vi "KEVIN GET USERS ITEMS.vi"(10 "BYU ID # IN":string, 11 "connection reference in":T3) -> (2 "DATA OUT":T2, 3 "connection reference out":T3)   [LabVIEW 2019]
uses:
  <vilib>/addons/database/Connection.llb/Conn ObjectReference.ctl
  Controls/Table Data Types/Inventory Data Type.ctl
  <vilib>/addons/database/Auxilliary.llb/DB Tools Cursor Type.ctl
  <vilib>/addons/database/Connection.llb/Conn Execute.vi
  <vilib>/addons/database/Recordset.llb/Rec Fetch Recordset Data (R).vi
  <vilib>/addons/database/Recordset.llb/Rec Destroy - Connection.vi
  <vilib>/addons/database/_DB Variant To Data/Database Variant To Data.xnode
  <vilib>/addons/database/NI_Database_API.lvlib
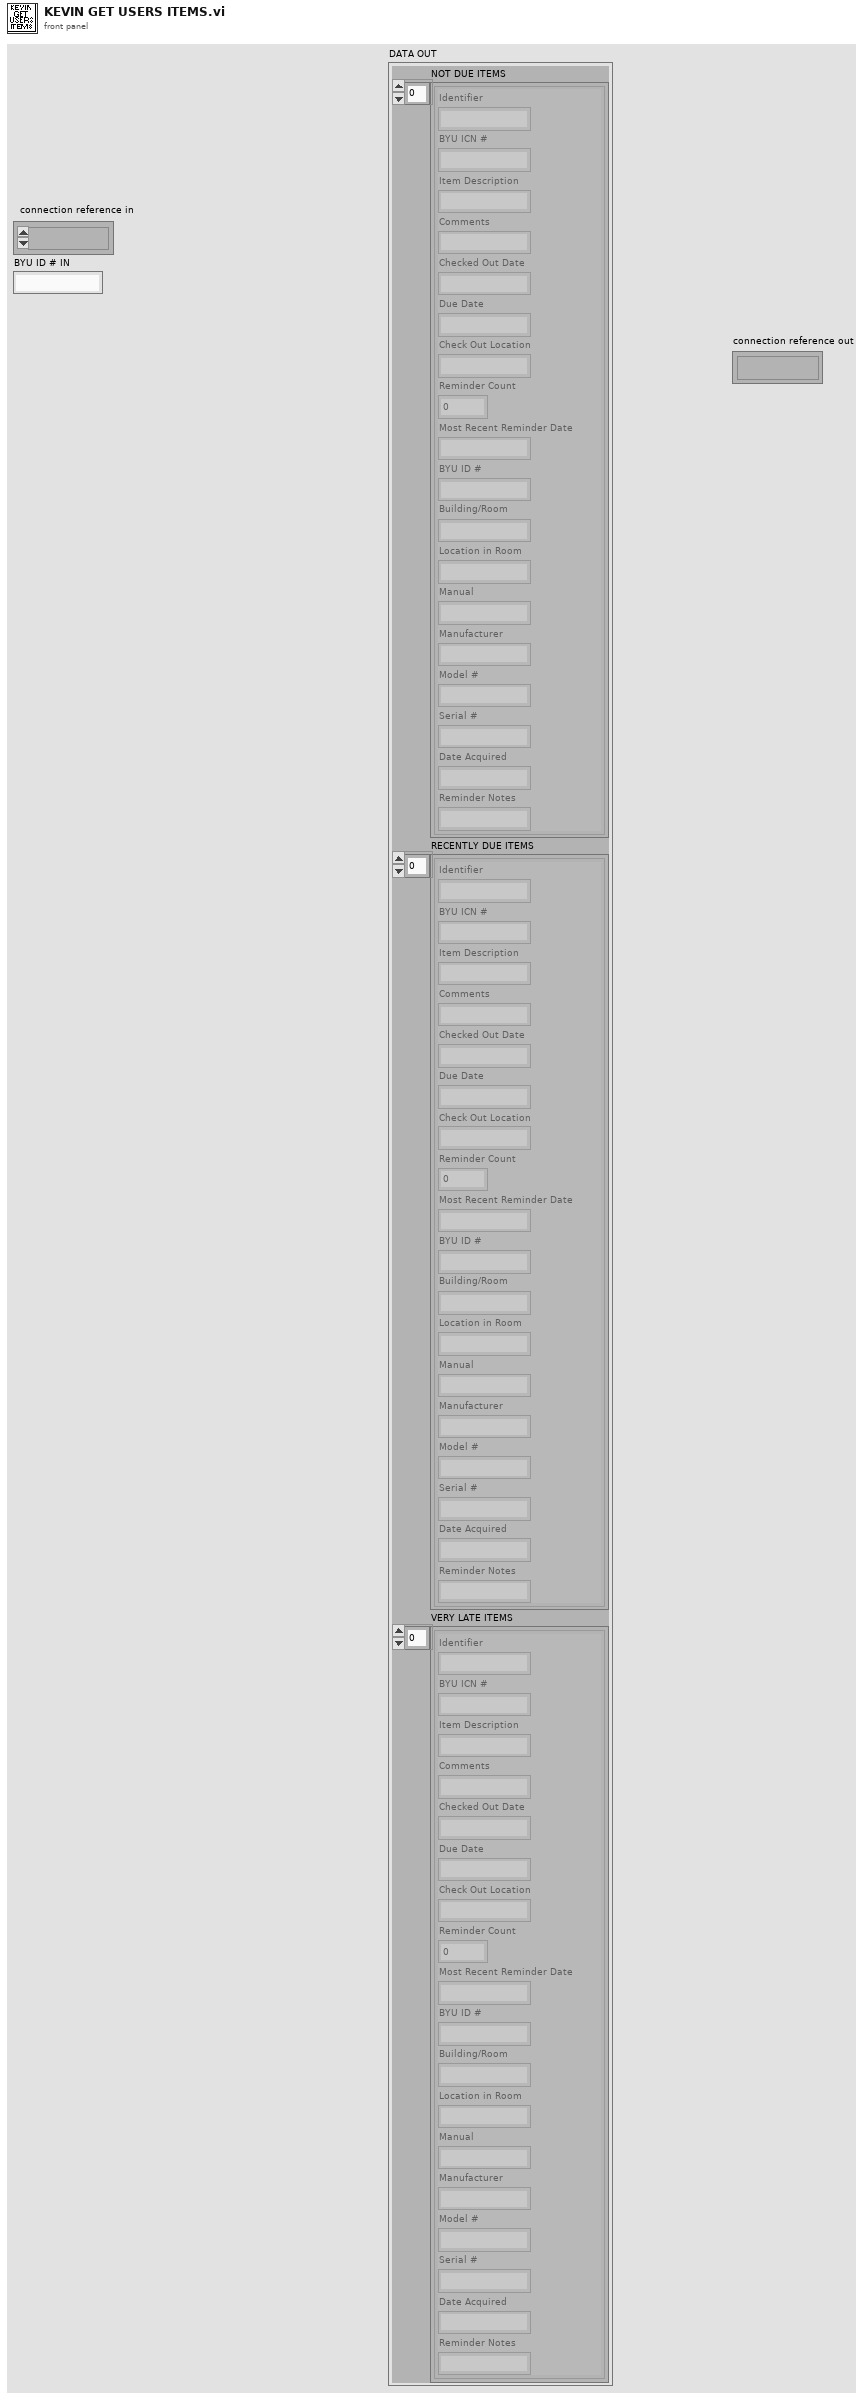
[diagram p1: front panel]
types:
  T1 = typedef "Inventory Data Type.ctl" = cluster{"Identifier":string, "BYU ICN #":string, "Item Description":string, "Comments":string, "Checked Out Date":string, "Due Date":string, "Check Out Location":string, "Reminder Count":i32, "Most Recent Reminder Date":string, "BYU ID #":string, "Building/Room":string, "Location in Room":string, "Manual":string, "Manufacturer":string, "Model #":string, "Serial #":string, "Date Acquired":string, "Reminder Notes":string}
  T2 = cluster{"NOT DUE ITEMS":T1[], "RECENTLY DUE ITEMS":T1[], "VERY LATE ITEMS":T1[]}
  T3 = typedef "NI_Database_API.lvlib/Conn ObjectReference.ctl" = refnum<k1>
  T4 = typedef "NI_Database_API.lvlib/DB Tools Cursor Type.ctl" = enum16{"forward-only", "keyset", "dynamic", "static"}
  T5 = typedef "NI_Database_API.lvlib/Rec ObjectReference.ctl" = refnum<k1>
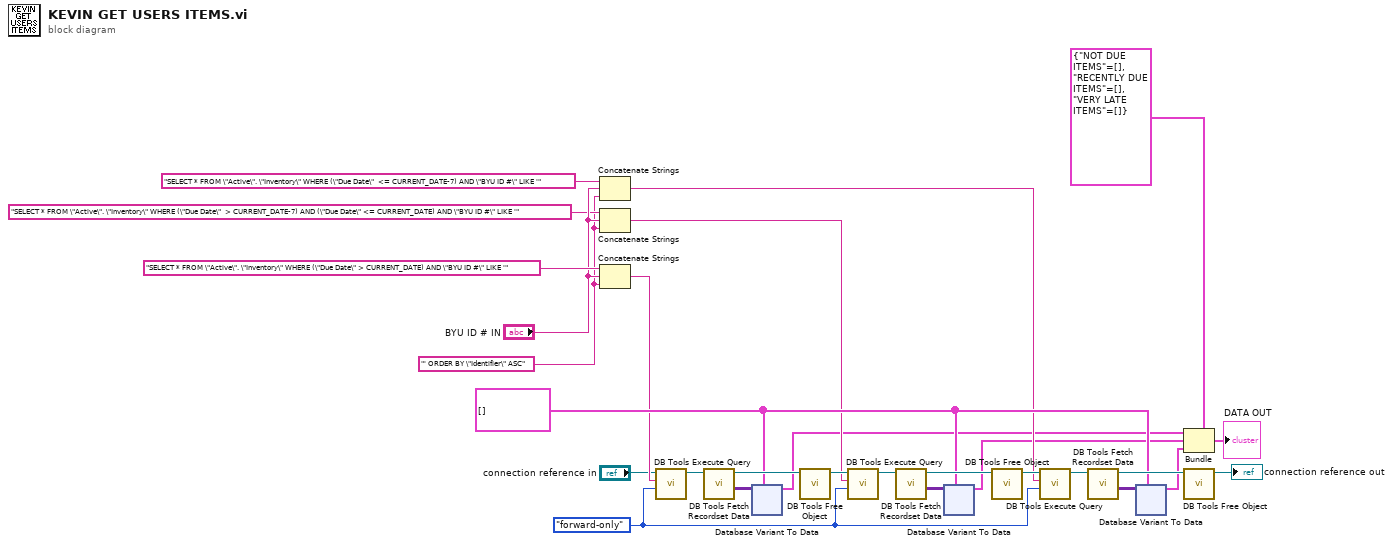
[diagram p0: block diagram]
diagram:
  w13 = DB_Tools_Cursor_Type."forward-only" ("cursor type")
  w7 = "' ORDER BY \"Identifier\" ASC"
  w15 = T1[] [] ("Array")
  n1 = Concatenate Strings("SELECT * FROM \"Active\". \"Inventory\" WHERE (\"Due Date\"  <= CURRENT_DATE-7) AND \"BYU ID #\" LIKE '", "BYU ID # IN", w7) -> (w11:string)
  n2 = Concatenate Strings("SELECT * FROM \"Active\". \"Inventory\" WHERE (\"Due Date\"  > CURRENT_DATE-7) AND (\"Due Date\" <= CURRENT_DATE) AND \"BYU ID #\" LIKE '", "BYU ID # IN", w7) -> (w12:string)
  n3 = Concatenate Strings("SELECT * FROM \"Active\". \"Inventory\" WHERE (\"Due Date\" > CURRENT_DATE) AND \"BYU ID #\" LIKE '", "BYU ID # IN", w7) -> (w14:string)
  n4 = call-poly <vilib>:"DB Tools Execute Query.vi"("cursor type"=w13, "SQL query"=w14, "connection reference"="connection reference in") -> ("recordset reference"=w24:T5)  [unwired: 5 in, 1 out]
  n5 = call-poly <vilib>:"DB Tools Fetch Recordset Data.vi"("recordset reference"=w24) -> ("recordset data"=w26:variant[][], "recordset reference out"=w25:T5)  [unwired: 4 in, 1 out]
  n6 = xnode "Database Variant To Data"("database variant"=w26, "type"=w15) -> ("data"=w4:T1[])  [unwired: 1 in, 1 out]
  n7 = call-poly <vilib>:"DB Tools Free Object.vi"("recordset reference"=w25) -> ("connection reference"=w20:T3)  [unwired: 9 in, 1 out]
  n8 = call-poly <vilib>:"DB Tools Execute Query.vi"("cursor type"=w13, "SQL query"=w12, "connection reference"=w20) -> ("recordset reference"=w23:T5)  [unwired: 5 in, 1 out]
  n9 = call-poly <vilib>:"DB Tools Fetch Recordset Data.vi"("recordset reference"=w23) -> ("recordset data"=w21:variant[][], "recordset reference out"=w22:T5)  [unwired: 4 in, 1 out]
  n10 = xnode "Database Variant To Data"("database variant"=w21, "type"=w15) -> ("data"=w3:T1[])  [unwired: 1 in, 1 out]
  n11 = call-poly <vilib>:"DB Tools Free Object.vi"("recordset reference"=w22) -> ("connection reference"=w16:T3)  [unwired: 9 in, 1 out]
  n12 = call-poly <vilib>:"DB Tools Execute Query.vi"("cursor type"=w13, "SQL query"=w11, "connection reference"=w16) -> ("recordset reference"=w17:T5)  [unwired: 5 in, 1 out]
  n13 = call-poly <vilib>:"DB Tools Fetch Recordset Data.vi"("recordset reference"=w17) -> ("recordset data"=w19:variant[][], "recordset reference out"=w18:T5)  [unwired: 4 in, 1 out]
  n14 = xnode "Database Variant To Data"("database variant"=w19, "type"=w15) -> ("data"=w2:T1[])  [unwired: 1 in, 1 out]
  n15 = Bundle(cluster=T2 {"NOT DUE ITEMS"=[], "RECENTLY DUE ITEMS"=[], "VERY LATE ITEMS"=[]} ("EMAIL ITEMS"), "NOT DUE ITEMS"=w4, "RECENTLY DUE ITEMS"=w3, "VERY LATE ITEMS"=w2) -> (→"DATA OUT":T2)
  n16 = call-poly <vilib>:"DB Tools Free Object.vi"("recordset reference"=w18) -> ("connection reference"=→"connection reference out":T3)  [unwired: 9 in, 1 out]
